vi "Create Trigger Model Dynamic Limit Branch.vi"(0 "VISA resource name":refnum<visa-resource-name>, 2 "Measurement Block":i32 min=1 format="%#.6g", 5 "Block Number (1)":i32 min=1 format="%#.6g", 7 "Limit Type":u16(ring) items=["Above", "Below", "Inside", "Outside"], 11 "error in (no error)":errorcluster, 12 "Branch To Block":i32 min=1 format="%#.6g") -> (4 "VISA resource name out":refnum<visa-resource-name>, 15 "error out":errorcluster)   [LabVIEW 2009, in "Keithley DMM7510.lvlib"]
doc: "This VI defines a trigger model block that goes to a specified block in the trigger model if a measurement meets user-defined criteria."
uses:
  Keithley DMM7510.lvlib
panel:
  in  "Limit Number":i32 min=1 max=2 step=1 format="%#.6g"
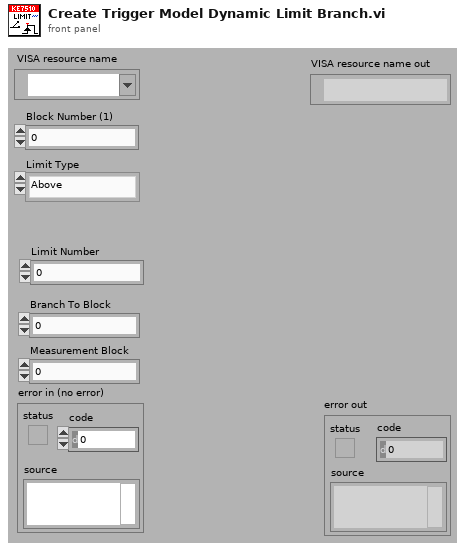
[diagram p1: front panel]
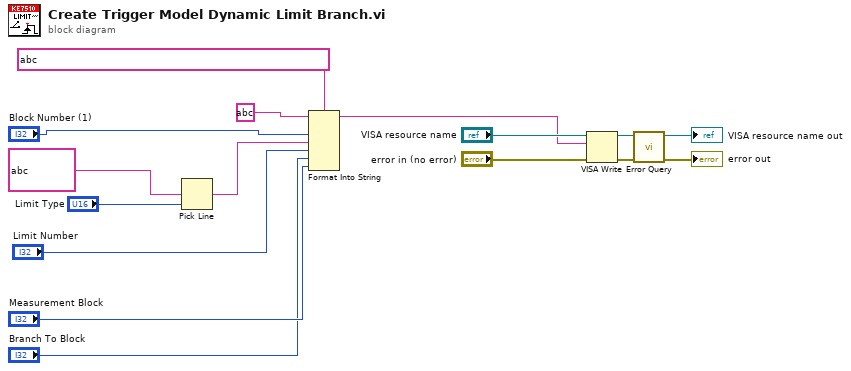
[diagram p0: block diagram]
diagram:
  n1 = Pick Line(multi-line string=string ?, line index="Limit Type") -> (output string=w6:string)  [unwired: 1 in]
  n2 = Format Into String(format string=string ?, initial string=string ?, "Block Number (1)", w6, "Limit Number", "Branch To Block", "Measurement Block") -> (resulting string=w8:string)  [unwired: 1 in, 1 out]
  n3 = VISA Write(VISA resource name="VISA resource name", write buffer=w8, error in (no error)="error in (no error)") -> (VISA resource name out=w12:refnum<visa-resource-name>, error out=w11:errorcluster)  [unwired: 1 out]
  n4 = call "Error Query.vi"("error in (no error)"=w11, "VISA resource name"=w12) -> ("error out"=→"error out":errorcluster, "VISA resource name out"=→"VISA resource name out":refnum<visa-resource-name>)  [unwired: 8 out]
